vi "Send Receive b.vi"(0 "Arduino Resource":T3, 5 "Data":u8[](array[numeric]), 7 "Bytes To Read (0)":u8, 9 "Time Out (100 ms)":i32=500, 11 "error in":errorcluster) -> (4 "Arduino Resource out":T3, 8 "Read Buffer":string, 15 "error out":errorcluster)   [LabVIEW 2015]
uses:
  <vilib>/LabVIEW Interface for Arduino/Type Defs/Board Type.ctl
  <vilib>/LabVIEW Interface for Arduino/Type Defs/Connection Type.ctl
  <vilib>/LabVIEW Interface for Arduino/LabVIEW Interface for Arduino.lvlib
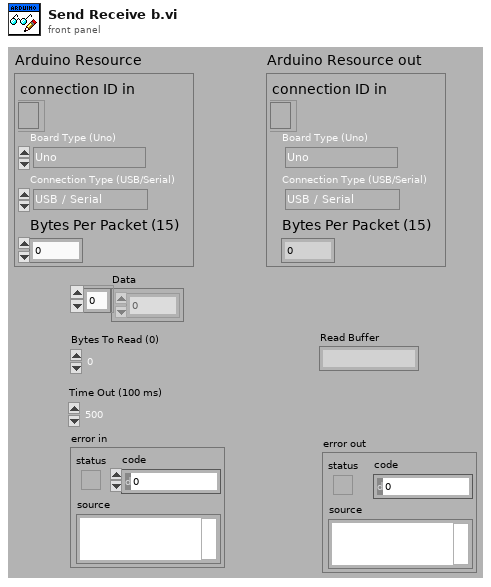
[diagram p1: front panel]
types:
  T1 = typedef "LabVIEW Interface for Arduino.lvlib/Board Type.ctl" = enum16{"Uno", "Dimuelanove w/Atmega 328", "Mega 2560"}
  T2 = typedef "LabVIEW Interface for Arduino.lvlib/Connection Type.ctl" = enum8{"USB / Serial", "XBEE", "BlueSmirf (Bluetooth)"}
  T3 = cluster{"connection ID in":refnum<k31>, "Board Type (Uno)":T1, "Connection Type (USB/Serial)":T2, "Bytes Per Packet (15)":u32}
  T4 = enum16{"Standard", "Buffered", "CRLF", "Immediate"}
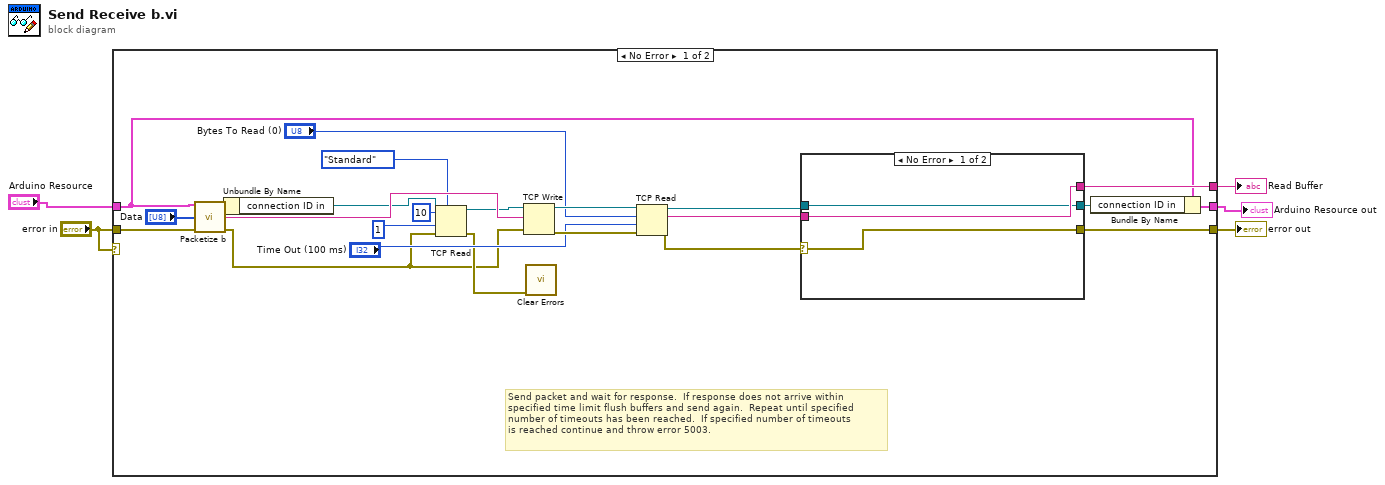
[diagram p0: block diagram]
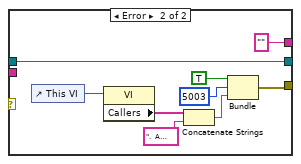
[diagram p2: hidden frame]
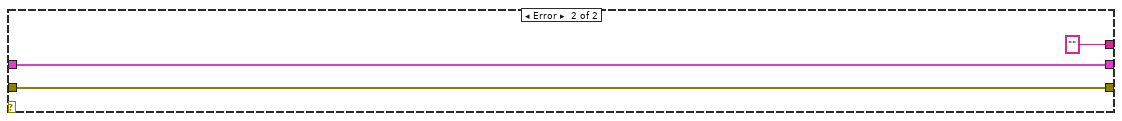
[diagram p3: hidden frame]
diagram:
  n1 = case shown="No Error" "error in" {
    tunnel: [w27 w41] -> w5
    tunnel: [w26 "" ("read buffer")] -> w4
    tunnel: "error in" -> [w25 w41]
    tunnel: "Arduino Resource" -> [w14 w42]
    tunnel: [w14 w42] -> w1
    frame No Error {
      # "Send packet and wait for response.  If response does not arrive within \nspecified time limit flush buffers and send again.  Repeat until specified \nnumber of timeouts has been reached.  If specified number of timeouts\nis reached continue and throw error 5003."
      n2 = call "Packetize b.vi"("Arduino Resource in"=w14, "Data"="Data", "error in"=w25) -> ("Arduino Resource out"=w22:T3, "Packet"=w23:string, "error out"=w7:errorcluster)  [unwired: 10 in]
      n3 = Unbundle By Name(w22) -> ("connection ID in"=w6:refnum<k31>)
      n4 = TCP Read(connection ID=w6, bytes to read=10, error in (no error)=w7, 7:T4."Standard" ("mode (standard)"), 9:1 ("timeout ms (25000)")) -> (connection ID out=w12:refnum<k31>, error out=w8:errorcluster)  [unwired: 1 out]
      n5 = TCP Write(connection ID=w12, data in=w23, error in (no error)=w7) -> (connection ID out=w21:refnum<k31>, error out=w20:errorcluster)  [unwired: 1 in, 1 out]
      n6 = call <vilib>:"Clear Errors.vi"("error in (no error)"=w8) -> ()  [unwired: 5 in, 2 out]
      n7 = TCP Read(connection ID=w21, bytes to read="Bytes To Read (0)", error in (no error)=w20, 9:"Time Out (100 ms)") -> (connection ID out=w17:refnum<k31>, data out=w16:string, error out=w18:errorcluster)  [unwired: 1 in]
      n8 = case shown="No Error" w18 {
        selector: w18 -> [w30 _]
        tunnel: [w30 w34] -> w27
        tunnel: [w29 "" ("read buffer")] -> w26
        tunnel: w17 -> [w28 w39]
        tunnel: [w28 w39] -> w15
        tunnel: w16 -> [w29 _]
        frame No Error {
        }
        frame Error {
          n9 = control-ref of="This VI"() -> (w35:refnum<vi>)
          n10 = property class="VI"(reference=w35) -> ("Callers"=w36:string[])  [unwired: 1 in, 2 out]
          n11 = Concatenate Strings(w36, ".  A timeout occurred while trying to read form the Arduino." ("string")) -> (w33:string)
          n12 = Bundle(TRUE, "code"=5003, w33) -> (w34:cluster{bool, "code":i32, string})  [unwired: 1 in]
        }
      }
      n13 = Bundle By Name(cluster=w14, "connection ID in"=w15) -> ()  [unwired: 1 out]
    }
    frame Error {
    }
  }
  "error out" <- w5
  "Read Buffer" <- w4
  "Arduino Resource out" <- w1
